vi "PID.vi"() -> ()   [LabVIEW 2011]
doc: "This example is a template that gives the structure of a single-loop PID controller. This VI uses the PID Filter VI to reduce measurement noise. This VI also uses the PID Autotuning VI to tune the controller based on the closed-loop response. This VI also uses the Timed Loop to ensure deterministic execution.\n\nReplace the Dummy Input and Dummy Output VIs with code that communicates with a real-time target."
uses:
  <vilib>/addons/Digital Filter Design/_Objects.llb/DFD Filter Obj.ctl
  <vilib>/addons/Digital Filter Design/_Objects.llb/DFD Filter Coef.ctl
  <vilib>/addons/Digital Filter Design/_Objects.llb/DFD Filter Structure Type Selector.ctl
  <vilib>/addons/Digital Filter Design/_Objects.llb/dfd_Internal Quantization Settings.ctl
  <vilib>/addons/Digital Filter Design/_Objects.llb/dfd_Internal Quantization Srcs.ctl
  <vilib>/addons/Digital Filter Design/_Objects.llb/DFD Coef Norm Type.ctl
  <vilib>/Platform/TimedLoop/XDataNode/timing_clust.ctl
  <vilib>/Platform/TimedLoop/XDataNode/nitl_modes.ctl
  <vilib>/Platform/TimedLoop/XDataNode/wakeup.ctl
  <vilib>/DAQmx/write.llb/DAQmx Write (Counter Frequency 1Chan 1Samp).vi
  <vilib>/DAQmx/write.llb/DAQmx Write (Digital 1D Bool NChan 1Samp 1Line).vi
  <vilib>/DAQmx/read.llb/DAQmx Read (Counter DBL 1Chan 1Samp).vi
  <vilib>/DAQmx/read.llb/DAQmx Read (Analog 1D DBL NChan 1Samp).vi
  <vilib>/addons/control/pid/pid.llb/PID Advanced (DBL Array).vi
  <vilib>/addons/control/pid/pid.llb/PID Derivative Action Buffered (DBL Array).vi
  <vilib>/addons/control/pid/pid.llb/PID Get Advanced Error (DBL Array).vi
  <vilib>/addons/control/pid/pid.llb/PID Integral Action Buffered (DBL Array).vi
  <vilib>/addons/control/pid/pid.llb/PID Resize 1D Array.vi
  <vilib>/addons/control/pid/pid.llb/PID Get Advanced Error (DBL).vi
  <vilib>/DAQmx/create/channels.llb/DAQmx Create Channel (CO-Pulse Generation-Frequency).vi
  <vilib>/DAQmx/configure/timing.llb/DAQmx Timing (Implicit).vi
  <vilib>/DAQmx/miscellaneous.llb/DAQmx Fill In Error Info.vi
  <vilib>/addons/Digital Filter Design/Process.llb/DFD Filtering (PtByPt NChan).vi
  <vilib>/addons/control/pid/pid.llb/PID Parameter Manager (DBL Array).vi
  <vilib>/Platform/TimedLoop/XDataNode/XDataNode.xnode
  <vilib>/Platform/TimedLoop/XDataNode/XDNodeRunTimeDep.lvlib
  <vilib>/addons/Digital Filter Design/NI_DigFilterLicensed.lvlib
  <vilib>/addons/control/pid/NI_PID_pid.lvlib
panel:
  in  "linearity":dbl=1.0 format="%.2f"
  out "PIDGainsOut":T1(array[cluster])=[{"proportional gain (Kc)"=0.30000000000000004, "integral time (Ti, min)"=0.0, "derivative time (Td, min)"=0.0}, {"proportional gain (Kc)"=0.30000000000000004, "integral time (Ti, min)"=0.0, "derivative time (Td, min)"=0.0}, {"proportional gain (Kc)"=0.30000000000000004, "integral time (Ti, min)"=0.0, "derivative time (Td, min)"=0.0}]
  in  "PIDGains":T2={"proportional high (Kc)"=0.5, "integral high (Ti, min)"=0.0, "derivative high (Td, min)"=0.0, "derivative low (Td, min)"=0.0, "integral low (Ti, min)"=0.0, "proportional low (Kc)"=0.1}
  in  "PWMFreq(Hz)":dbl=20000.0 format="%#.6f"
  out "EncMax":dbl[](array[numeric])=[6.498, 6.518000000000001, 6.474]
  in  "BndrsCluster":T3={"InwardLimit(%)"=[0.7, 0.7, 0.7], "OutwardLimit(%)"=[0.3, 0.3, 0.3], "SpringCnst"=[5.0, 5.0, 5.0]}
  out "EncPos":dbl[](array[numeric])=[5.53125, 5.478, 5.5135000000000005]
  out "LP_LoadCell":T4={"mSRate_Fs"=500.0, "mSRate_Version"="2.0", "mSRate_Comments"="", "mSRate_OrgCoef"={"type"=enum."IIR Cascaded Second Order Sections Form II Transposed", "gain"=1.0, "coef a (k)"=[-0.36952737735124136, 0.1958157126558331], "coef b (v)"=[0.20657208382614797, 0.41314416765229595, 0.20657208382614797]}, "mSRate_CurCoef"={"type"=enum."IIR Cascaded Second Order Sections Form II Transposed", "gain"=1.0, "coef a (k)"=[-0.36952737735124136, 0.1958157126558331], "coef b (v)"=[0.20657208382614797, 0.41314416765229595, 0.20657208382614797]}, "mSRate_Quantized?"=FALSE, "mSRate_QCoef"={"type"=enum."Undefined", "gain"=1.0, "coef a (k)"=[], "coef b (v)"=[]}, "mSRate_QSettings"=[], "mSRate_Order"=2, "mSRate_Scaling"={"mSRate_ScaleByPowerOf2?"=FALSE, "mSRate_ScaleType"=enum."No Norm"}} {"mSRate_QSettings"."source" items=["Coef a/k"=0, "Coef b/v"=7, "Input"=1, "Output"=2, "Multiplicand"=3, "Product"=4, "Sum"=5, "Delay"=6, "Gain"=8]}
  in  "LP_LoadCell(Hz)":dbl=100.0
  out "MotorDir":bool[](array[boolean])=[FALSE, TRUE, TRUE]
  in  "ChartLength":dbl=2000.0
  out "FFTArray":dbl[](array[numeric])=[0.09102094165909652, 0.08880080695999211, 0.08742537267011773, 0.08903439623636634, 0.09196169234838143, 0.09470367128274114, 0.09783665070128943, 0.09789838144314505, 0.09594205914249723, 0.09363339103027582, 0.09111500840178702, 0.09203831504284742, 0.09713069022987347, 0.10134606515787001, 0.10061861907733752, 0.09843897276856389, 0.09804067529312961, 0.09755044051782759, 0.0976403166754025, 0.09725636922533248, 0.09471411781510511, 0.09289638367605484, 0.09463637756896869, 0.10108862118124308, 0.10335985683317359, 0.09643477655571013, 0.09248787564173953, 0.09323062466464398, 0.09304905947987505, 0.09264978533169155, 0.09214417573397773, 0.09390841780702704, 0.09540399956340267, 0.09227373877182224, 0.09095729107756384, 0.09392871530582937, 0.0943702886709022, 0.08818127732286983, 0.0807007270500169, 0.08222546366236534, 0.09239407386402292, 0.10311749567286, 0.10471285762085267, 0.0964395109898104, 0.09034274660193076, 0.08915833478556265, 0.08816672057416365, 0.09132499663965439, 0.09827291267684694, 0.1000111309712641, 0.0980408243845543, 0.09529649141150409, 0.09168769480452336, 0.09175909791948443, 0.09571722605296652, 0.10078396610263962, 0.10337942605788164, 0.1014243160339357, 0.0973879688812122, 0.09262209630248038, 0.09031450404738024, 0.09331444243965803, 0.09853176609365545, 0.09611436535238259, 0.0883462084018524, 0.09316531134912277, 0.10558468641824159, 0.10678886347597229, 0.09760830011954734, 0.09111787329777818, 0.0897474453433214, 0.09177388258440985, 0.09614267796476492, 0.09981294892553577, 0.10684721226661176, 0.1078320930394148, 0.0968659399944411, 0.0925416262100675, 0.10030149307473206, 0.10238166455529184, 0.09521176688144757, 0.09585474281406252, 0.10141419849985543, 0.10250775879644676, 0.10131637786742215, 0.09823895961308332, 0.09987441648394499, 0.10271171935070175, 0.09869498899095455, 0.09802502865960976, 0.1013086559148363, 0.09767917025294583, 0.0903655011057841, 0.08830538594258142, 0.09119640016394422, 0.09324595223234786, 0.0945781693605675, 0.0961364777205373, 0.0973689435310479, 0.0981906075001171, 0.09650428184662667, 0.09320201923696174, 0.09218527453800356, 0.0928641968506453, 0.08880772620180627, 0.08549814225091175, 0.0918160400789082, 0.09924044045331475, 0.1006880024780284, 0.09709457652728365, 0.09175252607866341, 0.08881311705339597, 0.08676962298788296, 0.08909276722465459, 0.09745872636630303, 0.10002363387018202, 0.09474941391798437, 0.09479589463639002, 0.10619301053989326, 0.11013974313018808, 0.09810776285710797, 0.09159224898156491, 0.09454586178729105, 0.09738746387133843, 0.09683758569714396, 0.09317703251887542, 0.09145502676796455, 0.09195341475060125, 0.09183726851232944, 0.09314903943899071, 0.09621764664922357, 0.10006496184605966, 0.1086383293940109, 0.11026483076134179, 0.09740502737526889, 0.08962730114947677, 0.09204878325853857, 0.0965956485415745, 0.09926388339064521, 0.09908199133688707, 0.10311544290730992, 0.10622108107448491, 0.10065490376453218, 0.09399221564191973, 0.09082253310177452, 0.09271102497698457, 0.1012525124499937, 0.10602868530341275, 0.1026722749787491, 0.10319758832877436, 0.1036662954376473, 0.09813164549595414, 0.09820127558939208, 0.09874362737972482, 0.09261795007496774, 0.0925548637284494, 0.09688408303332961, 0.0931475786261286, 0.0874255261985941, 0.08857582919835429, 0.09211457350330834, 0.09393722111205698, 0.09662856411913412, 0.10123111196606292, 0.10296596776556342, 0.09836056791312328, 0.09235906685147227, 0.09028608175232539, 0.09426437771841292, 0.1001298758773979, 0.10379001436697999, 0.10384108815645533, 0.09815350124546153, 0.09463245337646703, 0.09495433061374936, 0.09248312317373729, 0.08821395727649654, 0.09073953337473195, 0.11323141000634579, 0.12885170155313352, 0.11310065142851995, 0.09769712603806086, 0.09064228954662149, 0.08669795029054495, 0.09082560583271858, 0.09294253567100298, 0.09080399783545823, 0.09192238471589097, 0.09646212722798142, 0.09897805347628216, 0.10431964577385561, 0.10970370530272601, 0.10447413729321658, 0.0959824501621602, 0.0937564320831249, 0.09555675083496182, 0.09843334250128712, 0.10010272181170206, 0.09739437719983716, 0.09394850769089175, 0.09312455120007386, 0.09252291619942024, 0.09219859129440382, 0.09330029323013085, 0.09635625418417197, 0.09989377979578923, 0.09707740950360141, 0.0825286400290957, 0.0742116515981123, 0.0835614097568316, 0.08967018271289941, 0.08809761919163403, 0.0899393812674251, 0.09601098267213592, 0.10044097204337782, 0.09885423777819236, 0.09531572484531821, 0.09436358572146161, 0.0950122057032307, 0.09464476199601543, 0.0947150937691509, 0.09536558141734598, 0.09589427668828288, 0.09526844145691217, 0.09206680991571439, 0.09024003039093455, 0.09227319889926314, 0.09694714177637125, 0.10013985115058632, 0.09927970382273595, 0.10003415571128227, 0.10652988935956782, 0.10576392054710738, 0.09458357237591669, 0.09132343408427156, 0.09539181733336558, 0.0983186064913613, 0.10242688312844601, 0.10440435360069594, 0.10006353383872878, 0.09603975944753498, 0.09566845237077003, 0.09445646943948487, 0.0937258427916497, 0.096498399173728, 0.09934752344549783, 0.0990571102573801, 0.09550810506979841, 0.09029380751494616, 0.09042573958060648, 0.09386549349043373, 0.09458778223341384, 0.10046364491796721, 0.10786347691619338, 0.10438883183150918, 0.09842565593409977, 0.09948204841067702, 0.10101784574352315, 0.09750221132446843, 0.09253571579725435, 0.08956807568195971, 0.08996922635990895, 0.09433244803273629, 0.0981400001262236, 0.09730951016555453, 0.09498002406290165, 0.09550454698949373, 0.09548292078434514, 0.09344281054064055, 0.09411914317897263, 0.09732202289260564, 0.09889327555577414, 0.09671120193041986, 0.09441990679723493, 0.09342686394131444, 0.091365411976931, 0.09050845132446485, 0.09534263430143414, 0.10306713778181106, 0.10450584487448797, 0.0990234509740975, 0.09084127256203062, 0.08709369142597481, 0.09021656273727405, 0.09181028260020982, 0.09109823283902471, 0.09044727443610756, 0.09251548654394454, 0.09736503986769181, 0.09901179246490464, 0.09671517642563755, 0.09518087378212874, 0.09586163678264449, 0.09648979737720542, 0.09725576734099747, 0.09719171821726084, 0.09723530353050332, 0.098663678328929, 0.09773982233939164, 0.09515580263043158, 0.09465776080429732, 0.09400629716840968, 0.09022515258196406, 0.08947371447551435, 0.09513694728563658, 0.09811254490785551, 0.09620635414337135, 0.09507651859514187, 0.0945267183869635, 0.09382421725979852, 0.0956459361826017, 0.09791579910376325, 0.09561349463035275, 0.09394343712503771, 0.09541610000519386, 0.09347644946854719, 0.0897683685757062, 0.0882604517220544, 0.08974524575043759, 0.09617177978036573, 0.10785004696265986, 0.11303390708229241, 0.10597687870653058, 0.10151283573345282, 0.1009344792379192, 0.09784368867081476, 0.09904071888600943, 0.10349669840280362, 0.1040942209998349, 0.10148782505936726, 0.09657490042623461, 0.09314115873421659, 0.09476689178493831, 0.09736746158346737, 0.09940753670154678, 0.10763997903819085, 0.11479529854711948, 0.1069768316687588, 0.09678246562153861, 0.09437403607619825, 0.08991926190075022, 0.08464072873932871, 0.0838422049156726, 0.08585411986322508, 0.09270974096714582, 0.09842968109345317, 0.09900983413969505, 0.0977284165379058, 0.09370619379559553, 0.09096138996160992, 0.0927353404991053, 0.09549410171143649, 0.09741545780358865, 0.09850179236874584, 0.09753334029902613, 0.0938944804227653, 0.09095421884359461, 0.09176025760176629, 0.09470966226615142, 0.09819729499972707, 0.10092611404338708, 0.10287110068670076, 0.1027962250137489, 0.0978173622830017, 0.09254050160889164, 0.09136446540164815, 0.09231575018234112, 0.09434223474076338, 0.09602581659968036, 0.09496820926423802, 0.09116816115664508, 0.08735998487494422, 0.08701165052963132, 0.0918752420339039, 0.09535937616272426, 0.09170292684335234, 0.08637152315549343, 0.09056762543199076, 0.10125595578883476, 0.10271469202300029, 0.09775950759891888, 0.09454609145608173, 0.09306695582041324, 0.09377828073481509, 0.09588077835169251, 0.0979142076883873, 0.09882700945913166, 0.09933648933168406, 0.099033187772869, 0.09653834537480366, 0.09303951793244071, 0.09170465830988545, 0.0941457996614852, 0.09809651341412748, 0.09818062942287485, 0.09582697341162467, 0.09876838394989043, 0.10546921279135386, 0.10275346946121104, 0.09194145449807363, 0.0898225988833451, 0.092125626983029, 0.09370523623585021, 0.09919143901749372, 0.1041951636993691, 0.1066806743004945, 0.10416052948131936, 0.09792099668505777, 0.0952797809377209, 0.09566488601699888, 0.09765147292508924, 0.10113211837654253, 0.10299017639955342, 0.10366729558308667, 0.10191018057912563, 0.09649506988129782, 0.09389071214465278, 0.09557003425213123, 0.09675362737028138, 0.09448731542418246, 0.09265805501182751, 0.09330679658333524, 0.09198404724267795, 0.09127001888440069, 0.09226181555741168, 0.09234502799301768, 0.09219260874297533, 0.09453712895651711, 0.10177796737055392, 0.10958340153225894, 0.10975413491769775, 0.10248466010004485, 0.09536732020150841, 0.09120648811873355, 0.09184800643569438, 0.0986821321253647, 0.10626473072965756, 0.10537453718446824, 0.09520288322362136, 0.08904581063864876, 0.09132773436696105, 0.09514741844304171, 0.09749575758565918, 0.09770635670783624, 0.09799993015447016, 0.09951651213649035, 0.0995205342643167, 0.09687835611906422, 0.09357010582888718, 0.0885918098064579, 0.08590153653140457, 0.09300058682888698, 0.10077446286178039, 0.09991133951530635, 0.09560751560574979, 0.091214169602366, 0.08723907760025741, 0.08892627554995633, 0.09644549844999885, 0.10032051369342253, 0.09912534271581792, 0.09915992139838321, 0.09921451306525575, 0.09778223224387768, 0.09717830735035844, 0.09588013614993547, 0.0927780200018827, 0.09185512397969973, 0.09542549643518046, 0.10008272634984831, 0.10116817181133533, 0.09777543290620841, 0.09466137486733109, 0.09592060890150078, 0.09823504847463188, 0.10058777942336122, 0.10237950070466754, 0.10291698250275211, 0.10768901733126822, 0.10885439884737656, 0.09993104128484098, 0.09276540111803068, 0.09186436245127866, 0.09278994548771279, 0.09166516641293293, 0.09228869480917856, 0.0971713653637861, 0.09912513860644213, 0.09791813921378399, 0.09619280883929195, 0.09366600704017955, 0.09261344714559394, 0.09503915956804532, 0.0981984537879128, 0.09992496692007144, 0.10029654314248054, 0.09863461151252964, 0.09767691053553712, 0.10129973257952882, 0.10181786448461859, 0.09380545602539495, 0.09166428615872282, 0.10000876289467604, 0.10461129330592896, 0.10091426652576975, 0.09590902708070043, 0.09107718711458933, 0.08849791000210501, 0.09200138898585147, 0.09615962040336506, 0.09800372498507702, 0.09893065057675744, 0.0983955647047802, 0.09876634377612285, 0.10151929001679223, 0.10142412979690257, 0.09873475610715217, 0.09890105704989277, 0.09902227746104335, 0.09874144041158964, 0.09929080648579931, 0.09700621727454077, 0.09396554312862367, 0.09411993528641702, 0.09805078929441152, 0.10094385557815756, 0.0995766211211698, 0.09716790672549175, 0.0931507383918105, 0.09005818765844088, 0.09047072972860055, 0.09209656254058018, 0.0913595214132443, 0.09083708412716954, 0.09633256393122286, 0.10087922683078064, 0.10007708228545206, 0.0964043140555525, 0.09289043553835055, 0.09278715599047352, 0.09355315634006024, 0.09450708646843198, 0.10020802674913763, 0.10439641118267241, 0.10017050640257566, 0.09696154696372317, 0.09856007457682515, 0.09758362764252046, 0.09301238360933117, 0.09208989460000822, 0.09535103523500486, 0.09704488040248786, 0.09649501624947075, 0.09292136947127232, 0.08762683169458144, 0.08807286018124134, 0.09251512532824335, 0.09352523022465763, 0.09482456898370897, 0.09857201880281713, 0.10002741623318949, 0.0992614963411499, 0.09819623421351308, 0.09500221408641796, 0.09101806214044308, 0.09063953610348258, 0.09294804769796418, 0.09618044842316048, 0.09864344832634965, 0.09731409098146067, 0.09275731640689558, 0.08958824930657339, 0.08921529543689591, 0.09008924014780986, 0.0922843798603982, 0.09366216208769575, 0.09558199939758943, 0.09828305461466146, 0.09595370732739364, 0.09169090724242437, 0.09486275276922365, 0.09918003470009631, 0.09588463863675534, 0.09615114899202093, 0.10736894176307686, 0.11426943369080936, 0.10533053641881585, 0.09160572246627915, 0.08553935463051385, 0.0881349187985328, 0.09242294313221106, 0.09337402639419164, 0.09331159712083947, 0.09479064404311334, 0.09484349059638743, 0.09248513554256084, 0.09116154660902528, 0.09085685038813406, 0.09296507129029936, 0.09815989027368009, 0.10195227362645769, 0.10228117738839224, 0.10085835473943733, 0.09751269602240561, 0.09370967555567532, 0.09308864653624445, 0.09809065792911877, 0.10390797237770644, 0.10428729986453797, 0.10484705321736316, 0.1063439573737108, 0.10359279242064043, 0.09924852703831326, 0.0952494758177389, 0.09358370667783035, 0.09489784057415311, 0.09501487632028198, 0.0949785525307149, 0.09702974980573481, 0.09938770889790986, 0.0998162055714144, 0.09843377911152251, 0.09703349670590405, 0.09737469105942545, 0.10041408832460698, 0.10236929336371704, 0.10038794849578446, 0.09549563254588557, 0.09230552912861477, 0.09428579109294094, 0.09733021192971705, 0.10009575535906687, 0.10063699551446069, 0.09840489572564667, 0.09822220083516732, 0.09670831294753654, 0.09206699400033341, 0.09171882085270323, 0.09472323262887117, 0.09469805184174276, 0.09561204111984363, 0.09882415494294253, 0.10089755073599155, 0.1009746372012849, 0.09800452889416644, 0.09404398605476502, 0.09018878155226688, 0.08785389300929711, 0.0892087878331425, 0.09349918860945793, 0.09875258866777097, 0.09728600636028967, 0.08773113491061649, 0.0856815303077994, 0.09392363414267457, 0.09684633020230474, 0.09423852280049147, 0.09341352749318232, 0.09226654402586368, 0.09227710107356496, 0.09271963202497929, 0.08942468552678305, 0.08808004412932355, 0.09082025208462184, 0.0943662584247623, 0.0986132484395693, 0.10278541971811173, 0.10425562139598878, 0.10338672407937001, 0.10069281462171725, 0.09461155564547581, 0.09043898221032887, 0.09086241811178179, 0.0956465654213487, 0.10047432523652337, 0.09874012995090306, 0.09662845273612478, 0.09742358901085837, 0.0954416126025474, 0.0944343225427322, 0.10061701780076883, 0.10282239184753347, 0.09680988544522648, 0.09594049942946489, 0.09952890382137601, 0.09851203949360546, 0.09321353268952194, 0.08874726896721062, 0.08937458303830566, 0.09502426723593145, 0.09704743909405683, 0.09341309909207127, 0.09320657330533846, 0.09541194900634187, 0.09621262807269083, 0.09597209460726519, 0.0948260222868175, 0.09694872112465212, 0.10544860150868023, 0.10962955571826748, 0.10094655844693746, 0.09411998258104398, 0.09602810074338575, 0.09644720495875421, 0.09428721442198901, 0.09214689947843446, 0.08792921462480895, 0.08716373336696479, 0.09197270134951673, 0.09204920268606104, 0.09073306300519976, 0.0939728839595127, 0.09356066685722333, 0.08812625530222079, 0.08846796813662568, 0.09920222450533496, 0.1058252143911878, 0.10188908820115482, 0.09868257472108143, 0.0974471506866546, 0.09586570959738368, 0.09545399635530576, 0.09528028923958379, 0.09603600268580659, 0.09766986117065025, 0.09961126326024015, 0.102743664979939, 0.1017975484717779, 0.09590417887737472, 0.09436986087302418, 0.0960950471893677, 0.09258002402887018, 0.09004428691053806, 0.09505743810555885, 0.09878514128365433, 0.10297684075522308, 0.10611677505693812, 0.10082620695105142, 0.09620687334027836, 0.09310800002970553, 0.09182827527750033, 0.095727744524222, 0.09705375327189339, 0.09458796542608221, 0.09301369005214323, 0.09210520432889652, 0.08993839931550959, 0.08913016197974472, 0.09255624228469467, 0.09975241664086784, 0.10670570585410949, 0.10549643336652603, 0.09861578062160453, 0.09146706187237587, 0.08594071806729495, 0.08518463683142836, 0.08854217583721581, 0.0956823300983743, 0.10118154007919228, 0.09853336945909529, 0.08922985179977319, 0.08315873460741482, 0.08728364339410201, 0.09516133282168092, 0.09881287906379264, 0.09672407737478446, 0.0921373488185896, 0.09041236841979136, 0.09121915468652697, 0.08966211275954464, 0.09075594338729104, 0.09907330650665794, 0.10137052776123553, 0.09380125383649235, 0.09394083443448777, 0.09991051836702212, 0.098914133127104, 0.09474091321489582, 0.09161425833149173, 0.0903816234241194, 0.09213408364075391, 0.09528216461959353, 0.09974635308501201, 0.10296376102767685, 0.09948494250957257, 0.09245409320787697, 0.0847234037653295, 0.08124359196979607, 0.08732159111454053, 0.09312453042992751, 0.09443572094409348, 0.09614806429690329, 0.09811827039050844, 0.09920582650164311, 0.09697117498814982, 0.0916159658944723, 0.0891856040590495, 0.09258576128000563, 0.09850595311479003, 0.10216466234193508, 0.10159404847792461, 0.09813734713893262, 0.09316946471982161, 0.089898245406245, 0.09143198123581918, 0.09608607140091953, 0.09873473423395897, 0.09694929148980345, 0.09669789085980723, 0.09956690918966572, 0.0977729875277695, 0.0923041238418928, 0.09046565059013356, 0.09216640295809489, 0.0959330768646728, 0.10013029478045048, 0.10036419805653103, 0.09737402883495548, 0.09529221761444011, 0.09474517102973008, 0.09517299304482099, 0.0970756321518759, 0.10255745875419961, 0.10794133323694724, 0.10505236763333477, 0.09758183404582535, 0.09518044092000434, 0.09686979136411433, 0.0963564439416678, 0.09593176854266736, 0.09809161877980843, 0.09924108473106583, 0.09921188778060949, 0.09940086043005295, 0.0975288291375136, 0.09337070989200846, 0.09236658901389715, 0.09472263130255579, 0.0968237224024725, 0.09996618180738043, 0.10162032330970641, 0.09956354926862832, 0.0977647659354574, 0.09604223038393135, 0.09382542241699236, 0.0933435847837743, 0.09628226322753937, 0.10836470695266869, 0.1185360866116867, 0.11067474781394153, 0.09722535798812948, 0.09059164647623978, 0.09037033981826824, 0.0922399309267108, 0.09078403611098936, 0.09105698636290141, 0.10376259966062101, 0.11649500331537674, 0.11130322578340691, 0.10170161330836708, 0.09786740170856437, 0.09448847841011596, 0.09104852113042589, 0.09094283375218719, 0.0954029276712423, 0.09824516819295355, 0.09849509459457706, 0.09973739131151854, 0.09774831102631165, 0.0927456448651611, 0.09108519344935982, 0.0920998105659684, 0.09434189366287797, 0.09780729946312651, 0.10036989043082956, 0.10109565912158552, 0.09515305577167105, 0.08736552269450357, 0.0884112935503377, 0.09177082542402804, 0.0941287855547005, 0.09738682229038303, 0.0986266391229788, 0.09859453485538511, 0.09729757794543303, 0.09535369697287284, 0.09491193402856518, 0.09415469374433652, 0.0919245995116571, 0.09260229053425066, 0.09711763046042896, 0.0994603212303976, 0.09848540559686833, 0.09555158263322422, 0.09193674661406673, 0.0912660558768004, 0.0918165368284526, 0.09254400827702049, 0.09586111175301713, 0.09772643877338094, 0.09347792465932281, 0.08884232697038624, 0.08922279597187947, 0.09187463167003444, 0.09629467739771397, 0.09992495848273909, 0.10084749495175446, 0.10510922114203466, 0.10708163951765005, 0.09956989395888909, 0.09332447144951299, 0.09340500283643924, 0.094880302503652, 0.09691342764719751, 0.09899058573507037, 0.09966082620027929, 0.0994892484004143, 0.09879975449547401, 0.09599706963028815, 0.09287049518749299, 0.09279118855764833, 0.0950213123437698, 0.09827611194296731, 0.10118169536703843, 0.10261122865414517, 0.10100060223624563, 0.09609561402187453, 0.09200743121302843, 0.08862116346806512, 0.08646433734107578, 0.09119532618246128, 0.09856972918486451, 0.10021442995888795, 0.09758803531006871, 0.09612123672642862, 0.09793415833895243, 0.09899538949715286, 0.09717460829930598, 0.09579196490738726, 0.09602730553486771, 0.09707847234544234, 0.09819997921636264, 0.09732600104331778, 0.09402548360669662, 0.09226028625168499, 0.09457498381103961, 0.10150378557624333, 0.11125041854722023, 0.11056373305326211, 0.0927818464378579, 0.08175411479726982, 0.08755354766678927, 0.0919741357023542, 0.0934579739365533, 0.09712071873894144, 0.09883277187119353, 0.09422826831892607, 0.09004330059339985, 0.09343182204109886, 0.09572244868720534, 0.09428955402912023, 0.09381445993796159, 0.09480061321748565, 0.09874815315489778, 0.10184085471542625, 0.0987270724155361, 0.09302194541720415, 0.08966533112846485, 0.08800933926523152, 0.08538174293270813, 0.08310551408863133, 0.0888319373985028, 0.10005332755264837, 0.10285518512108545, 0.09873141222733123, 0.0953230356843207, 0.09364591903170218, 0.09362054859116155, 0.09466451600736198, 0.09642449020644978, 0.09916989069119003, 0.10215644387012379, 0.10226405616775242, 0.09876434432117011, 0.09330880795867115, 0.09103536825394845, 0.09626304699088227, 0.10584964653613375, 0.10913250641565027, 0.10441438464989818, 0.10184381876786906, 0.09934814040303097, 0.09485819401222303, 0.09369531581738759, 0.0971066747794125, 0.11050198317269021, 0.1170005254963874, 0.10569386990870762, 0.09940418548326989, 0.09738145361344645]
  in  "LoopFreq(Hz)":dbl=500.0 caption="Set Loop Period (us)"
  in  "SetPoint":dbl[](array[numeric])=[5.0, 5.0, 5.0] min=-10.0 max=10.0 step=1.0
  out "PWMTaskC":refnum<k21>
  out "PWMTaskB":refnum<k21>
  in  "PIDLimit":dbl=0.5 caption="MaxDutyCycle" min=0.0 max=1.0 step=0.01 format="%.2f"
  out "LoopPeriod(s)":dbl=0.002 caption="Loop Period (s)" format="%#_10g"
  out "PWMTaskA":refnum<k21>
  out "LoopDuration(us)":i64=1027 caption="Actual Loop Period (us)"
  in  "stop":bool
  out "SlowLoop":bool
  out "Graph":T10(graph)={7.024469067405356, "SetPointOut"=0.08674999999999766, "output"=0.09102094165909652, "output"=0.01281282497729658}
  # "Use to set force (limits = -10 to 10 lbs)"
  # "index"
  # "middle"
  # "thumb"
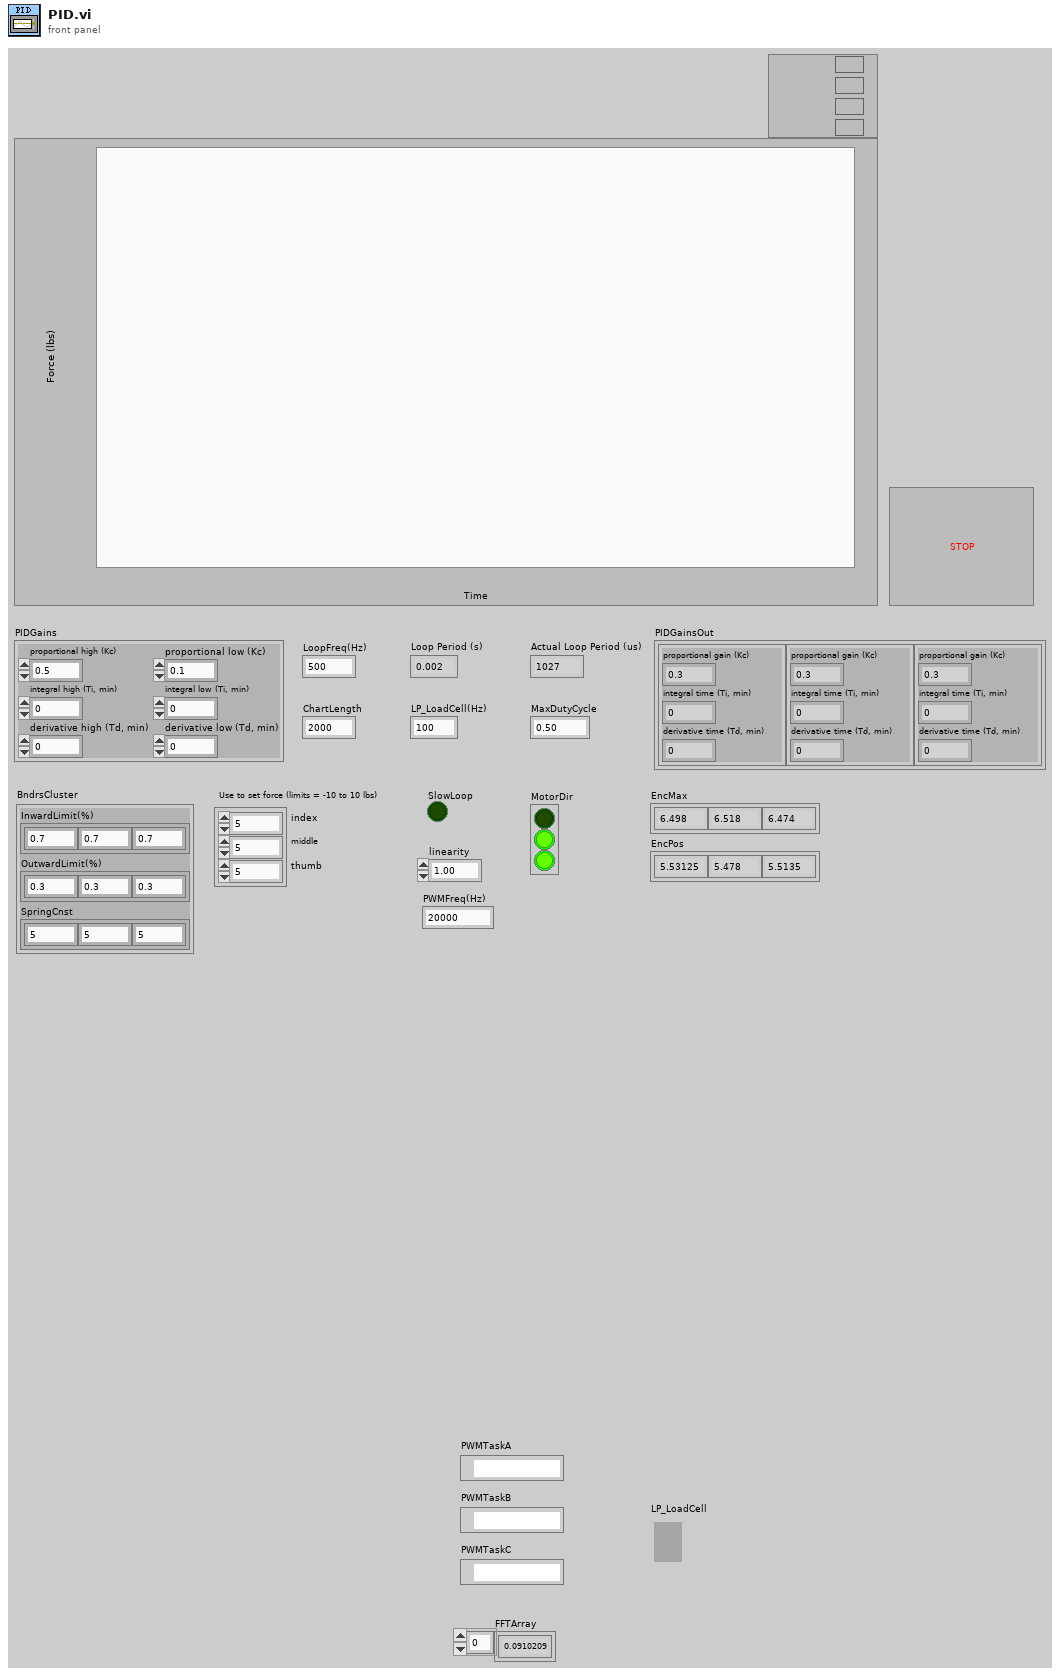
[diagram p1: front panel]
types:
  T1 = cluster{"proportional gain (Kc)":dbl, "integral time (Ti, min)":dbl, "derivative time (Td, min)":dbl}[]
  T2 = cluster{"proportional high (Kc)":dbl, "integral high (Ti, min)":dbl, "derivative high (Td, min)":dbl, "derivative low (Td, min)":dbl, "integral low (Ti, min)":dbl, "proportional low (Kc)":dbl}
  T3 = cluster{"InwardLimit(%)":dbl[], "OutwardLimit(%)":dbl[], "SpringCnst":dbl[]}
  T4 = typedef "NI_DigFilterLicensed.lvlib/DFD Filter Obj.ctl" = cluster{"mSRate_Fs":dbl, "mSRate_Version":string, "mSRate_Comments":string, "mSRate_OrgCoef":T5, "mSRate_CurCoef":T5, "mSRate_Quantized?":bool, "mSRate_QCoef":T5, "mSRate_QSettings":T7[], "mSRate_Order":i32, "mSRate_Scaling":cluster{"mSRate_ScaleByPowerOf2?":bool, "mSRate_ScaleType":T9}}
  T5 = typedef "NI_DigFilterLicensed.lvlib/DFD Filter Coef.ctl" = cluster{"type":T6, "gain":dbl, "coef a (k)":dbl[], "coef b (v)":dbl[]}
  T6 = typedef "NI_DigFilterLicensed.lvlib/DFD Filter Structure Type Selector.ctl" = enum16{"Undefined", "FIR Direct Form", "FIR Direct Form Transposed", "FIR Symmetric", "FIR Antisymmetric", "IIR Direct Form I", "IIR Direct Form I Transposed", "IIR Direct Form II", "IIR Direct Form II Transposed", "IIR Cascaded Second Order Sections Form I", "IIR Cascaded Second Order Sections Form I Transposed", "IIR Cascaded Second Order Sections Form II", "IIR Cascaded Second Order Sections Form II Transposed", "Lattice Allpass (basic sections)", "Lattice Allpass (one multiplier sections)", "Lattice Allpass (normalized sections)", "Lattice AR (basic sections)", "Lattice AR (one multiplier sections)", "Lattice AR (normalized sections)", "Lattice MA (minimum phase)", "Lattice MA (maximum phase)", "Lattice ARMA (basic sections)", "Lattice ARMA (one multiplier sections)", "Lattice ARMA (normalized sections)"}
  T7 = typedef "NI_DigFilterLicensed.lvlib/dfd_Internal Quantization Settings.ctl" = cluster{"source":T8, "wl":i16, "iwl":i16, "overflow mode":enum16{"Saturation", "Wrap"}, "rounding mode":enum16{"Nearest", "Truncation"}, "signed?":bool}
  T8 = typedef "NI_DigFilterLicensed.lvlib/dfd_Internal Quantization Srcs.ctl" = u16
  T9 = typedef "NI_DigFilterLicensed.lvlib/DFD Coef Norm Type.ctl" = enum16{"No Norm", "Time Domain 1-Norm", "Time Domain 2-Norm", "Time Domain Inf-Norm"}
  T10 = cluster{dbl, "SetPointOut":dbl, "output":dbl, "output":dbl}
  T11 = enum16{"Lowpass", "Highpass", "Bandpass", "Bandstop"}
  T12 = typedef "XDNodeRunTimeDep.lvlib/timing_clust.ctl" = cluster{"Expected End [f-1]":u64, "Actual End [f-1]":u64, "Finished Late? [f-1]":bool, "Expected End [i-1]":u64, "Actual End [i-1]":u64, "Finished Late? [i-1]":bool, "Expected Start [i]":u64, "Actual Start [i]":u64, "Expected Start [f]":u64, "Actual Start [f]":u64, "Source Name":string, "Structure Name":string, "Period":i64, "Deadline":i64, "Offset":i64, "Start":i64, "Priority":i32, "Timeout":i32, "Mode":T13, "Wakeup Reason":T14, "Error":errorcluster, "Source Type":string, "Secondary Source Type":string, "Global End Time":u64, "Global Start Time":u64, "Frame Duration":u64, "Iteration Duration":u64, "Assigned CPU":i32, "I/O Scan Engine Mode":u32}
  T13 = typedef "XDNodeRunTimeDep.lvlib/nitl_modes.ctl" = enum32{"No Change", "Process missed periods, maintain original phase", "Discard missed periods, maintain original phase", "Process missed periods, ignore original phase", "Discard missed periods, ignore original phase"}
  T14 = typedef "XDNodeRunTimeDep.lvlib/wakeup.ctl" = enum32{"Normal", "Aborted", "Asynchronous wakeup", "Timing source error", "Timed loop error", "Timeout"}
  T15 = cluster{"element":dbl, "element":dbl, "element":dbl, "element":dbl}
  T16 = cluster{"element":dbl, "element":dbl, "element":dbl, "element":dbl}[]
  T17 = cluster{"data":dbl, "SetPointIn":dbl, "Numeric":dbl, dbl}
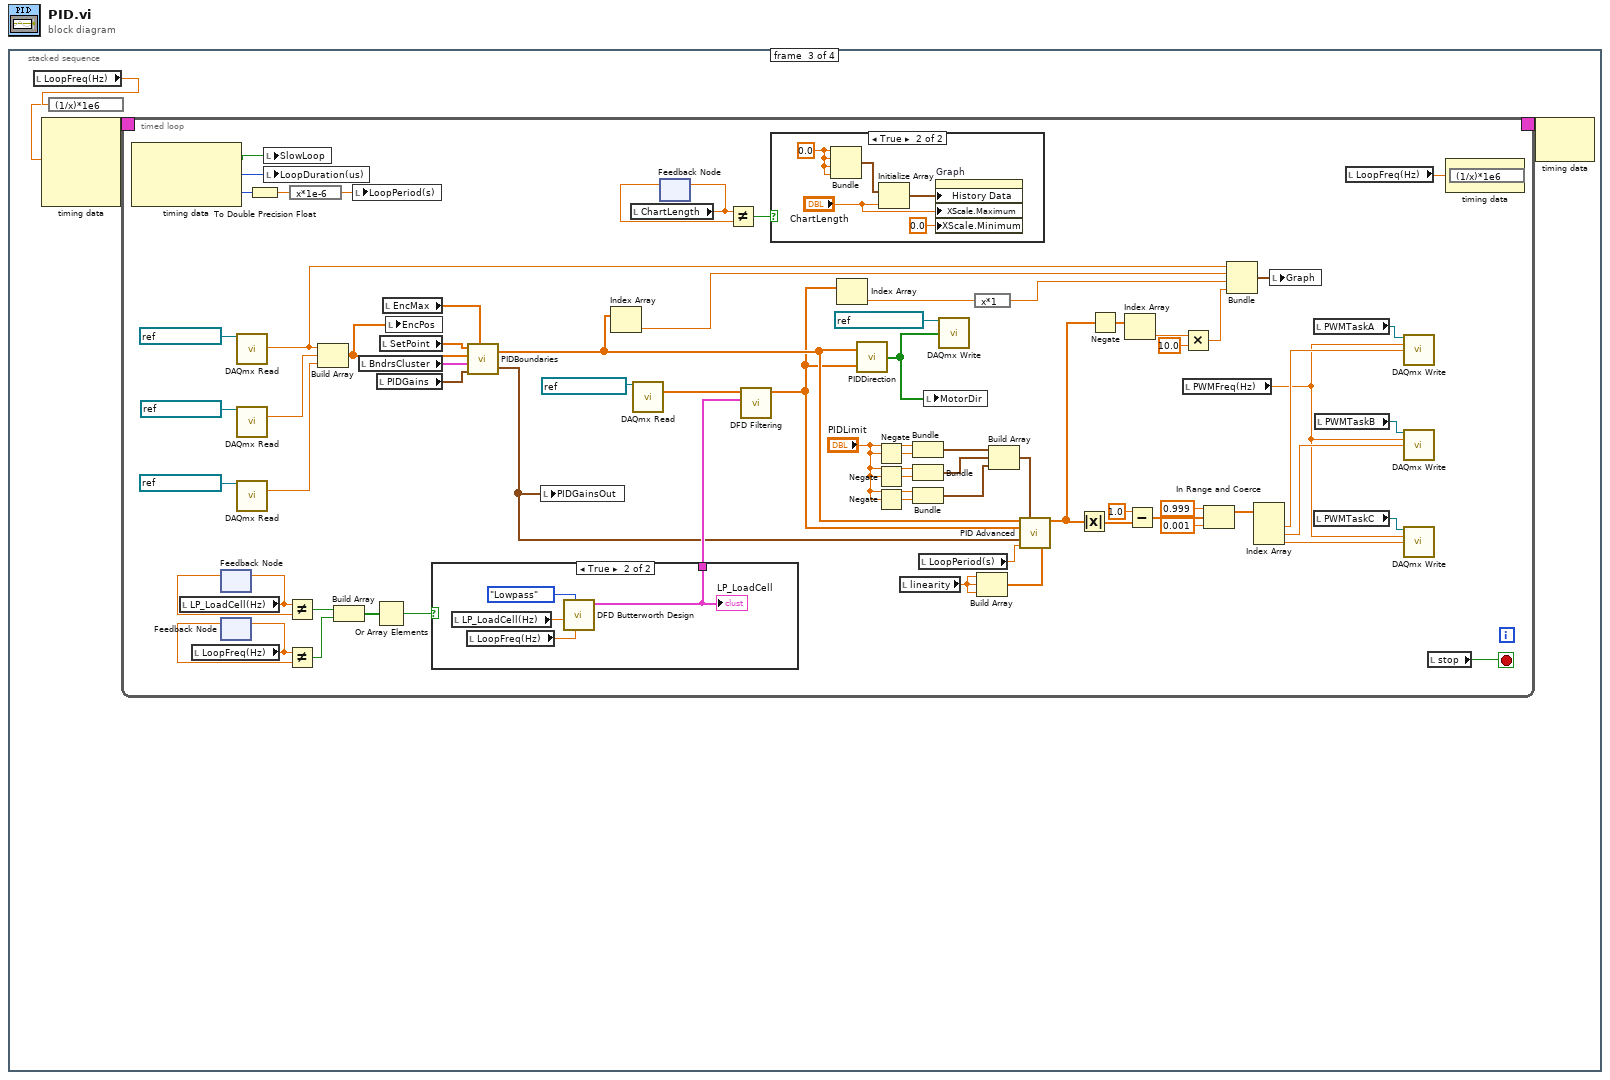
[diagram p0: block diagram]
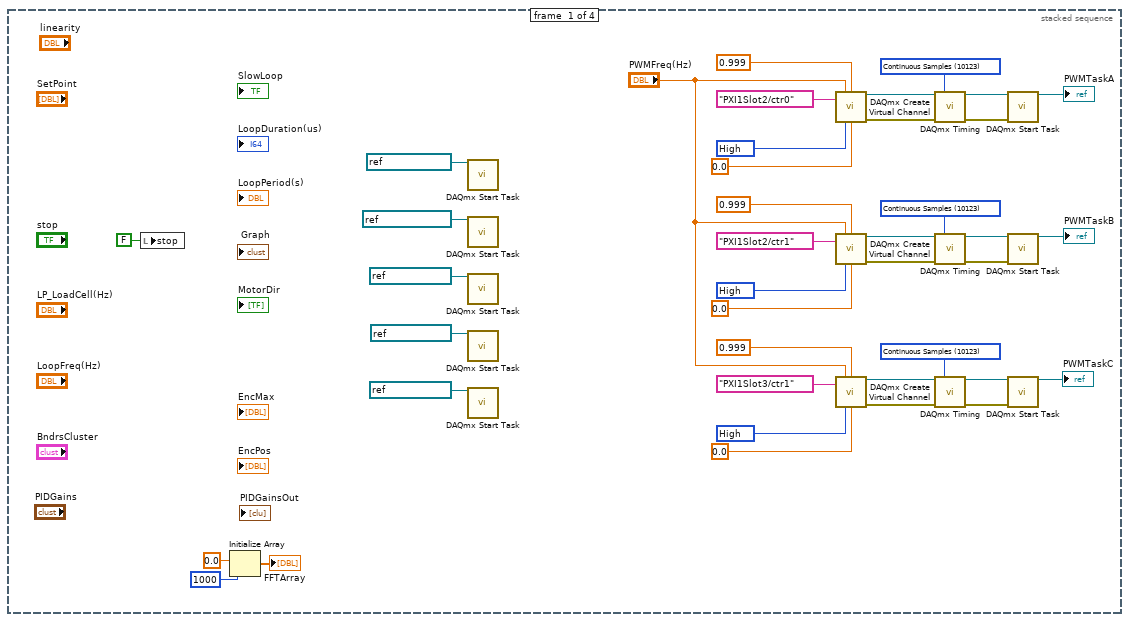
[diagram p2: hidden frame]
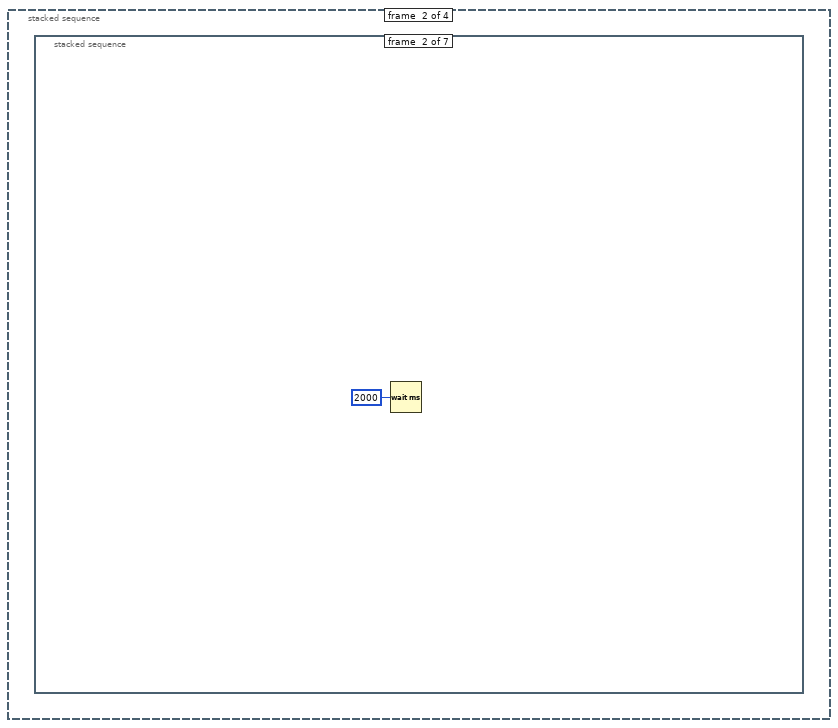
[diagram p3: hidden frame]
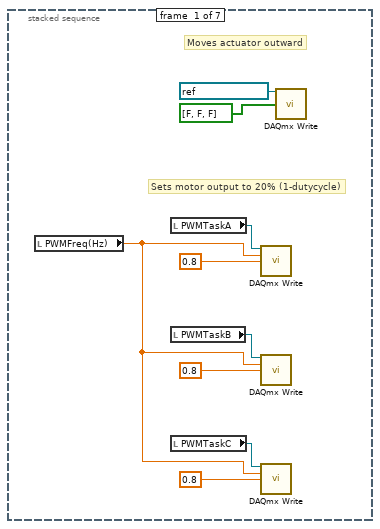
[diagram p4: hidden frame]
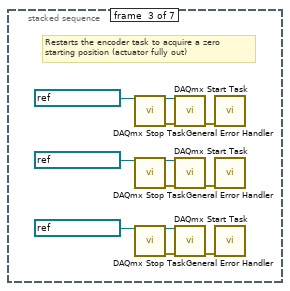
[diagram p5: hidden frame]
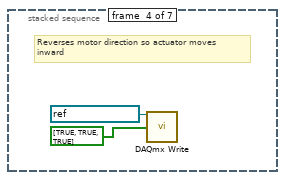
[diagram p6: hidden frame]
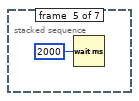
[diagram p7: hidden frame]
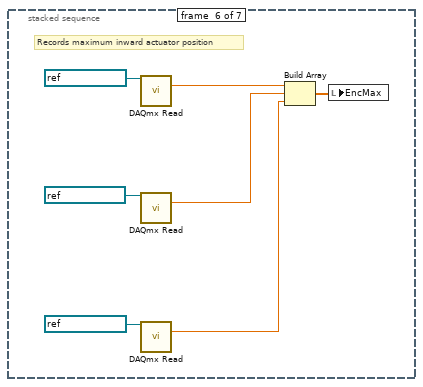
[diagram p8: hidden frame]
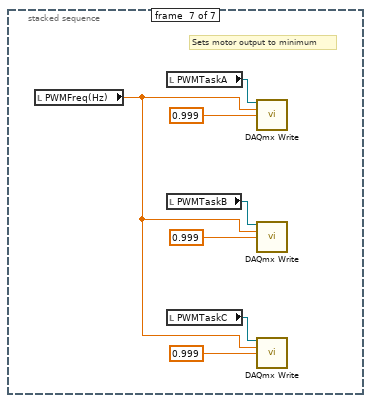
[diagram p9: hidden frame]
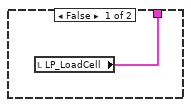
[diagram p11: hidden frame]
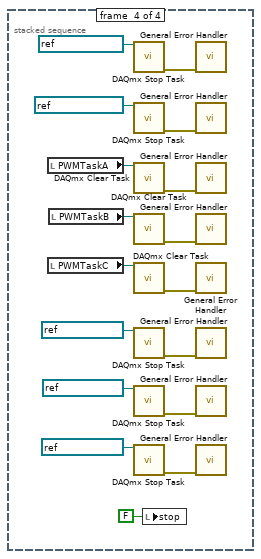
[diagram p12: hidden frame]
diagram:
  n1 = stacked-sequence {
    frame #0 {
      w10 = 10192 items=["High"=10192, "Low"=10214] ("idle state")
      w4 = 10123 items=["Finite Samples"=10178, "Continuous Samples"=10123] ("sample mode")
      w20 = 10192 items=["High"=10192, "Low"=10214] ("idle state")
      w26 = 10123 items=["Finite Samples"=10178, "Continuous Samples"=10123] ("sample mode")
      w37 = 10192 items=["High"=10192, "Low"=10214] ("idle state")
      w30 = 10123 items=["Finite Samples"=10178, "Continuous Samples"=10123] ("sample mode")
      n2 = local write "stop"(FALSE ("stop")) -> ()
      n3 = Initialize Array(0.0, 1000 ("dimension size")) -> (→"FFTArray":dbl[])
      n4 = call <vilib>:"DAQmx Start Task.vi"("task/channels in"=refnum<k21> "ForceInABC") -> ()  [unwired: 13 in, 2 out]
      n5 = call <vilib>:"DAQmx Start Task.vi"("task/channels in"=refnum<k21> "MotorDirABC") -> ()  [unwired: 13 in, 2 out]
      n6 = call <vilib>:"DAQmx Start Task.vi"("task/channels in"=refnum<k21> "PositionInA") -> ()  [unwired: 13 in, 2 out]
      n7 = call <vilib>:"DAQmx Start Task.vi"("task/channels in"=refnum<k21> "PositionInB" ("task")) -> ()  [unwired: 13 in, 2 out]
      n8 = call <vilib>:"DAQmx Start Task.vi"("task/channels in"=refnum<k21> "PositionInC") -> ()  [unwired: 13 in, 2 out]
      n9 = call-poly <vilib>:"DAQmx Create Virtual Channel.vi"("frequency"="PWMFreq(Hz)", "duty cycle"=0.999, "counter"=tag "PXI1Slot2/ctr0", "idle state"=w37, "initial delay"=0.0) -> ("task out"=w33:refnum<k21>, "error out"=w34:errorcluster)  [unwired: 9 in]
      n10 = call-poly <vilib>:"DAQmx Create Virtual Channel.vi"("frequency"="PWMFreq(Hz)", "duty cycle"=0.999, "counter"=tag "PXI1Slot2/ctr1", "idle state"=w20, "initial delay"=0.0) -> ("task out"=w23:refnum<k21>, "error out"=w22:errorcluster)  [unwired: 9 in]
      n11 = call-poly <vilib>:"DAQmx Create Virtual Channel.vi"("frequency"="PWMFreq(Hz)", "duty cycle"=0.999, "counter"=tag "PXI1Slot3/ctr1", "idle state"=w10, "initial delay"=0.0) -> ("task out"=w7:refnum<k21>, "error out"=w8:errorcluster)  [unwired: 9 in]
      n12 = call-poly <vilib>:"DAQmx Timing.vi"("task/channels in"=w33, "sample mode"=w30, "error in"=w34) -> ("task out"=w31:refnum<k21>, "error out"=w32:errorcluster)  [unwired: 11 in]
      n13 = call-poly <vilib>:"DAQmx Timing.vi"("task/channels in"=w23, "sample mode"=w26, "error in"=w22) -> ("task out"=w25:refnum<k21>, "error out"=w24:errorcluster)  [unwired: 11 in]
      n14 = call-poly <vilib>:"DAQmx Timing.vi"("task/channels in"=w7, "sample mode"=w4, "error in"=w8) -> ("task out"=w5:refnum<k21>, "error out"=w6:errorcluster)  [unwired: 11 in]
      n15 = call <vilib>:"DAQmx Start Task.vi"("task/channels in"=w31, "error in"=w32) -> ("task out"=→"PWMTaskA":refnum<k21>)  [unwired: 12 in, 1 out]
      n16 = call <vilib>:"DAQmx Start Task.vi"("task/channels in"=w25, "error in"=w24) -> ("task out"=→"PWMTaskB":refnum<k21>)  [unwired: 12 in, 1 out]
      n17 = call <vilib>:"DAQmx Start Task.vi"("task/channels in"=w5, "error in"=w6) -> ("task out"=→"PWMTaskC":refnum<k21>)  [unwired: 12 in, 1 out]
    }
    frame #1 {
      n18 = stacked-sequence {
        frame #0 {
          # "Sets motor output to 20% (1-dutycycle)"
          # "Moves actuator outward"
          n19 = local read "PWMFreq(Hz)"() -> (w41:dbl)
          n20 = local read "PWMTaskA"() -> (w48:refnum<k21>)
          n21 = local read "PWMTaskB"() -> (w45:refnum<k21>)
          n22 = local read "PWMTaskC"() -> (w42:refnum<k21>)
          n23 = call-poly <vilib>:"DAQmx Write.vi"("task/channels in"=w48, "frequency"=w41, "duty cycle"=0.8) -> ()  [unwired: 10 in, 3 out]
          n24 = call-poly <vilib>:"DAQmx Write.vi"("task/channels in"=w45, "frequency"=w41, "duty cycle"=0.8) -> ()  [unwired: 10 in, 3 out]
          n25 = call-poly <vilib>:"DAQmx Write.vi"("task/channels in"=w42, "frequency"=w41, "duty cycle"=0.8) -> ()  [unwired: 10 in, 3 out]
          n26 = call-poly <vilib>:"DAQmx Write.vi"("task/channels in"=refnum<k21> "MotorDirABC", "data"=bool[] [FALSE, FALSE, FALSE]) -> ()  [unwired: 11 in, 3 out]
        }
        frame #1 {
          n27 = Wait (ms)(milliseconds to wait=u32 2000) -> ()  [unwired: 1 out]
        }
        frame #2 {
          # "Restarts the encoder task to acquire a zero\nstarting position (actuator fully out)"
          n28 = call <vilib>:"DAQmx Stop Task.vi"("task/channels in"=refnum<k21> "PositionInA") -> ("task out"=w60:refnum<k21>, "error out"=w59:errorcluster)  [unwired: 13 in]
          n29 = call <vilib>:"DAQmx Stop Task.vi"("task/channels in"=refnum<k21> "PositionInB") -> ("task out"=w57:refnum<k21>, "error out"=w58:errorcluster)  [unwired: 13 in]
          n30 = call <vilib>:"DAQmx Stop Task.vi"("task/channels in"=refnum<k21> "PositionInC") -> ("task out"=w52:refnum<k21>, "error out"=w51:errorcluster)  [unwired: 13 in]
          n31 = call <vilib>:"DAQmx Start Task.vi"("task/channels in"=w60, "error in"=w59) -> ("error out"=w62:errorcluster)  [unwired: 12 in, 1 out]
          n32 = call <vilib>:"DAQmx Start Task.vi"("task/channels in"=w57, "error in"=w58) -> ("error out"=w55:errorcluster)  [unwired: 12 in, 1 out]
          n33 = call <vilib>:"DAQmx Start Task.vi"("task/channels in"=w52, "error in"=w51) -> ("error out"=w54:errorcluster)  [unwired: 12 in, 1 out]
          n34 = call <vilib>:"General Error Handler.vi"("error in (no error)"=w62) -> ()  [unwired: 10 in, 5 out]
          n35 = call <vilib>:"General Error Handler.vi"("error in (no error)"=w55) -> ()  [unwired: 10 in, 5 out]
          n36 = call <vilib>:"General Error Handler.vi"("error in (no error)"=w54) -> ()  [unwired: 10 in, 5 out]
        }
        frame #3 {
          # "Reverses motor direction so actuator moves\ninward"
          n37 = call-poly <vilib>:"DAQmx Write.vi"("task/channels in"=refnum<k21> "MotorDirABC", "data"=bool[] [TRUE, TRUE, TRUE]) -> ()  [unwired: 11 in, 3 out]
        }
        frame #4 {
          n38 = Wait (ms)(milliseconds to wait=u32 2000) -> ()  [unwired: 1 out]
        }
        frame #5 {
          # "Records maximum inward actuator position"
          n39 = call-poly <vilib>:"DAQmx Read.vi"("task/channels in"=refnum<k21> "PositionInA") -> ("data"=w69:dbl)  [unwired: 12 in, 2 out]
          n40 = call-poly <vilib>:"DAQmx Read.vi"("task/channels in"=refnum<k21> "PositionInB") -> ("data"=w68:dbl)  [unwired: 12 in, 2 out]
          n41 = call-poly <vilib>:"DAQmx Read.vi"("task/channels in"=refnum<k21> "PositionInC") -> ("data"=w67:dbl)  [unwired: 12 in, 2 out]
          n42 = Build Array(w69, w68, w67) -> (w66:dbl[])
          n43 = local write "EncMax"(w66) -> ()
        }
        frame #6 {
          # "Sets motor output to minimum"
          n44 = local read "PWMFreq(Hz)"() -> (w73:dbl)
          n45 = local read "PWMTaskA"() -> (w78:refnum<k21>)
          n46 = local read "PWMTaskB"() -> (w77:refnum<k21>)
          n47 = local read "PWMTaskC"() -> (w74:refnum<k21>)
          n48 = call-poly <vilib>:"DAQmx Write.vi"("task/channels in"=w78, "frequency"=w73, "duty cycle"=0.999) -> ()  [unwired: 10 in, 3 out]
          n49 = call-poly <vilib>:"DAQmx Write.vi"("task/channels in"=w77, "frequency"=w73, "duty cycle"=0.999) -> ()  [unwired: 10 in, 3 out]
          n50 = call-poly <vilib>:"DAQmx Write.vi"("task/channels in"=w74, "frequency"=w73, "duty cycle"=0.999) -> ()  [unwired: 10 in, 3 out]
        }
      }
    }
    frame #2 {
      n51 = local read "LoopFreq(Hz)"() -> (w81:dbl)
      n52 = expression code="(1/x)*1e6"(w81) -> (w80:dbl)
      n53 = node-c288(w80) -> (w83:T12)  [unwired: 3 in]
      n54 = timed-loop {
        timing: w83 -> [_]
        timing-out: [_] -> w82
        stop <- w131 stop-if-true
        n55 = node-c288() -> (w133:bool, w132:i64, w106:i64)  [unwired: 1 in]
        n56 = local read "LP_LoadCell(Hz)"() -> (w127:dbl)
        n57 = local read "LoopFreq(Hz)"() -> (w117:dbl)
        n58 = feedback #1() -> (w126:dbl)  [unwired: 1 in]
        n59 = feedback-in #1(w127) -> ()
        n60 = feedback #2() -> (w118:dbl)  [unwired: 1 in]
        n61 = feedback-in #2(w117) -> ()
        n62 = call-poly <vilib>:"DAQmx Read.vi"("task/channels in"=refnum<k21> "PositionInA") -> ("data"=w84:dbl)  [unwired: 12 in, 2 out]
        n63 = call-poly <vilib>:"DAQmx Read.vi"("task/channels in"=refnum<k21> "PositionInB") -> ("data"=w111:dbl)  [unwired: 12 in, 2 out]
        n64 = call-poly <vilib>:"DAQmx Read.vi"("task/channels in"=refnum<k21> "PositionInC") -> ("data"=w110:dbl)  [unwired: 12 in, 2 out]
        n65 = To Double Precision Float(number=w106) -> (double precision float=w105:dbl)
        n66 = local write "SlowLoop"(w133) -> ()
        n67 = local write "LoopDuration(us)"(w132) -> ()
        n68 = Not Equal?(x=w127, y=w126) -> (x != y?=w116:bool)
        n69 = Not Equal?(x=w117, y=w118) -> (x != y?=w115:bool)
        n70 = expression code="x*1e-6"(w105) -> (w119:dbl)
        n71 = Build Array(w84, w111, w110) -> (w107:dbl[])
        n72 = Build Array(w116, w115) -> (w114:bool[])
        n73 = local write "LoopPeriod(s)"(w119) -> ()
        n74 = local read "BndrsCluster"() -> (w103:T3)
        n75 = Or Array Elements(Boolean array=w114) -> (logical OR=w113:bool)
        n76 = local read "PIDGains"() -> (w96:T2)
        n77 = local read "SetPoint"() -> (w104:dbl[])
        n78 = local read "EncMax"() -> (w88:dbl[])
        n79 = local write "EncPos"(w107) -> ()
        n80 = case shown="True" w113 {
          tunnel: [w160 w161] -> w112
          frame False {
            n81 = local read "LP_LoadCell"() -> (w160:T4)
          }
          frame True {
            n82 = local read "LP_LoadCell(Hz)"() -> (w162:dbl)
            n83 = local read "LoopFreq(Hz)"() -> (w163:dbl)
            n84 = call <vilib>:"DFD Butterworth Design.vi"("fs [Hz]"=w163, "filter type"=T11."Lowpass", "low cutoff freq [Hz]"=w162) -> ("filter out"=w161:T4)  [unwired: 7 in, 1 out]
            "LP_LoadCell" <- w161
          }
        }
        n85 = call "PIDBoundaries.vi"("SetPointIn"=w104, "EncPosIn"=w107, "BndrsCluster"=w103, "PIDGainsIn"=w96, "EncMax"=w88) -> ("SetPointOut"=w109:dbl[], "PIDGainsOut"=w95:T1)
        n86 = local write "PIDGainsOut"(w95) -> ()
        n87 = Index Array(array=w109) -> (element=w108:dbl)  [unwired: 1 in]
        n88 = local read "ChartLength"() -> (w124:dbl)
        n89 = call-poly <vilib>:"DAQmx Read.vi"("task/channels in"=refnum<k21> "ForceInABC") -> ("data"=w94:dbl[])  [unwired: 12 in, 2 out]
        n90 = feedback #3() -> (w123:dbl)  [unwired: 1 in]
        n91 = feedback-in #3(w124) -> ()
        n92 = Not Equal?(x=w124, y=w123) -> (x != y?=w125:bool)
        n93 = call-poly <vilib>:"DFD Filtering.vi"("filter"=w112, "signal in"=w94) -> ("signal out"=w85:dbl[])  [unwired: 2 in, 7 out]
        n94 = case shown="True" w125 {
          frame False {
          }
          frame True {
            w155 = 0.0 ("element")
            n95 = Bundle("element"=w155, "element"=w155, "element"=w155, "element"=w155) -> (w159:T15)  [unwired: 1 in]
            n96 = Initialize Array(w159, "ChartLength") -> (w156:T16)
            n97 = property on="Graph" class="WFChart (strict)"("History Data"=w156, "XScale.Maximum"="ChartLength", "XScale.Minimum"=0.0 ("X Scale.Range:Minimum")) -> ()  [unwired: 2 in, 2 out]
          }
        }
        n98 = Index Array(array=w85) -> (element=w87:dbl)  [unwired: 1 in]
        n99 = call "PIDDirection.vi"("LoadCellIn"=w85, "SetPointIn"=w109) -> ("MotorDirOut"=w120:bool[])
        n100 = Negate(x="PIDLimit") -> (-x=w146:dbl)
        n101 = Negate(x="PIDLimit") -> (-x=w143:dbl)
        n102 = Negate(x="PIDLimit") -> (-x=w142:dbl)
        n103 = local read "linearity"() -> (w93:dbl)
        n104 = Bundle("PIDLimit"="PIDLimit", w146) -> (w141:cluster{"PIDLimit":dbl, dbl})  [unwired: 1 in]
        n105 = Bundle("PIDLimit"="PIDLimit", w143) -> (w140:cluster{"PIDLimit":dbl, dbl})  [unwired: 1 in]
        n106 = Bundle("PIDLimit"="PIDLimit", w142) -> (w139:cluster{"PIDLimit":dbl, dbl})  [unwired: 1 in]
        n107 = local read "LoopPeriod(s)"() -> (w129:dbl)
        n108 = local write "MotorDir"(w120) -> ()
        n109 = call-poly <vilib>:"DAQmx Write.vi"("task/channels in"=refnum<k21> "MotorDirABC", "data"=w120) -> ()  [unwired: 11 in, 3 out]
        n110 = expression code="x*1"(w87) -> (w86:dbl)
        n111 = Build Array(w93, w93, w93) -> (w92:dbl[])
        n112 = Build Array(w141, w140, w139) -> (w130:cluster{"PIDLimit":dbl, dbl}[])
        n113 = call-poly <vilib>:"PID Advanced.vi"("setpoint"=w109, "output range"=w130, "process variable"=w85, "PID gains"=w95, "dt (s)"=w129, "linearity"=w92) -> ("output"=w100:dbl[])  [unwired: 8 in, 1 out]
        n114 = Absolute Value(x=w100) -> (abs(x)=w128:dbl[])
        n115 = Negate(x=w100) -> (-x=w98:dbl[])
        n116 = Index Array(array=w98) -> (element=w91:dbl)  [unwired: 1 in]
        n117 = Subtract(x=1.0 ("y"), y=w128) -> (x-y=w152:dbl[])
        n118 = Multiply(x=w91, y=10.0) -> (x*y=w90:dbl)
        n119 = local read "PWMFreq(Hz)"() -> (w99:dbl)
        n120 = In Range and Coerce(upper limit=0.999, x=w152, lower limit=0.001) -> (coerced(x)=w137:dbl[])  [unwired: 1 out]
        n121 = Bundle("data"=w84, "SetPointIn"=w108, "Numeric"=w86, w90) -> (w97:T17)  [unwired: 1 in]
        n122 = Index Array(array=w137) -> (element #1=w136:dbl, element #2=w135:dbl, element #3=w134:dbl)  [unwired: 3 in]
        n123 = local write "Graph"(w97) -> ()
        n124 = local read "PWMTaskA"() -> (w147:refnum<k21>)
        n125 = local read "PWMTaskC"() -> (w121:refnum<k21>)
        n126 = local read "PWMTaskB"() -> (w145:refnum<k21>)
        n127 = local read "LoopFreq(Hz)"() -> (w102:dbl)
        n128 = call-poly <vilib>:"DAQmx Write.vi"("task/channels in"=w147, "frequency"=w99, "duty cycle"=w136) -> ()  [unwired: 10 in, 3 out]
        n129 = call-poly <vilib>:"DAQmx Write.vi"("task/channels in"=w145, "frequency"=w99, "duty cycle"=w135) -> ()  [unwired: 10 in, 3 out]
        n130 = call-poly <vilib>:"DAQmx Write.vi"("task/channels in"=w121, "frequency"=w99, "duty cycle"=w134) -> ()  [unwired: 10 in, 3 out]
        n131 = local read "stop"() -> (w131:bool)
        n132 = expression code="(1/x)*1e6"(w102) -> (w101:dbl)
        n133 = node-c288(w101) -> ()  [unwired: 1 out]
      }
      n134 = node-c288(w82) -> ()  [unwired: 1 out]
    }
    frame #3 {
      n135 = local read "PWMTaskA"() -> (w186:refnum<k21>)
      n136 = local read "PWMTaskC"() -> (w178:refnum<k21>)
      n137 = local read "PWMTaskB"() -> (w184:refnum<k21>)
      n138 = call <vilib>:"DAQmx Stop Task.vi"("task/channels in"=refnum<k21> "ForceInABC") -> ("error out"=w189:errorcluster)  [unwired: 13 in, 1 out]
      n139 = call <vilib>:"DAQmx Stop Task.vi"("task/channels in"=refnum<k21> "MotorDirABC") -> ("error out"=w190:errorcluster)  [unwired: 13 in, 1 out]
      n140 = call <vilib>:"DAQmx Clear Task.vi"("task in"=w186) -> ("error out"=w191:errorcluster)  [unwired: 14 in]
      n141 = call <vilib>:"DAQmx Clear Task.vi"("task in"=w184) -> ("error out"=w183:errorcluster)  [unwired: 14 in]
      n142 = call <vilib>:"DAQmx Clear Task.vi"("task in"=w178) -> ("error out"=w179:errorcluster)  [unwired: 14 in]
      n143 = call <vilib>:"DAQmx Stop Task.vi"("task/channels in"=refnum<k21> "PositionInA") -> ("error out"=w192:errorcluster)  [unwired: 13 in, 1 out]
      n144 = call <vilib>:"DAQmx Stop Task.vi"("task/channels in"=refnum<k21> "PositionInB") -> ("error out"=w181:errorcluster)  [unwired: 13 in, 1 out]
      n145 = call <vilib>:"DAQmx Stop Task.vi"("task/channels in"=refnum<k21> "PositionInC") -> ("error out"=w177:errorcluster)  [unwired: 13 in, 1 out]
      n146 = local write "stop"(FALSE ("stop")) -> ()
      n147 = call <vilib>:"General Error Handler.vi"("error in (no error)"=w189) -> ()  [unwired: 10 in, 5 out]
      n148 = call <vilib>:"General Error Handler.vi"("error in (no error)"=w190) -> ()  [unwired: 10 in, 5 out]
      n149 = call <vilib>:"General Error Handler.vi"("error in (no error)"=w191) -> ()  [unwired: 10 in, 5 out]
      n150 = call <vilib>:"General Error Handler.vi"("error in (no error)"=w183) -> ()  [unwired: 10 in, 5 out]
      n151 = call <vilib>:"General Error Handler.vi"("error in (no error)"=w179) -> ()  [unwired: 10 in, 5 out]
      n152 = call <vilib>:"General Error Handler.vi"("error in (no error)"=w192) -> ()  [unwired: 10 in, 5 out]
      n153 = call <vilib>:"General Error Handler.vi"("error in (no error)"=w181) -> ()  [unwired: 10 in, 5 out]
      n154 = call <vilib>:"General Error Handler.vi"("error in (no error)"=w177) -> ()  [unwired: 10 in, 5 out]
    }
  }
